vi "TagDB Refresh UI Value.vi"() -> ()   [LabVIEW 2017]
uses:
  2ef29265-346b-4d57-9e06-764a04e9d281.vi
  f314512e-c22b-4d02-bdf1-59be9bdd757c.vi
  22528161-74fa-4c81-9678-da9be87c1aa3.vi
  8fbe6154-e4cc-4ea5-b8fc-074bb6443d9f.vi
  f2742c4f-3dd1-44df-a39f-d6b0d834631b.vi
  922adba5-6730-477c-a9a6-f6ae257f51b2.vi
  c4b4571f-6e89-4cba-b3ba-78e7cbfa36bb.vi
  TagDB/_Support/DataAccess/data-Write.vi
  TagDB/_Support/Error/_[error50000]Invalid DB REF.vi
  TagDB/_Support/DataAccess/TagDB Ref to DVR.vi
  TagDB/_Support/DataAccess/_NameCacher.vi
  TagDB/_Support/Error/_[error50002]Invalid DataType.vi
  TagDB/_Support/URL/TRIM-BOTH-SPACE.vi
  TagDB/_Support/DataAccess/_datatypeChecker.vi
  <vilib>/Utility/Data Type/Get Type Information.vi
  TagDB/_Support/Error/_Build Error Cluster.vi
  TagDB/TagDB.lvlib
panel:
  in  "Update Period(ms)":u32(slide)=100 scale=1.0..1000.0
  out "String":string
  out "Numeric":dbl
  in  "stop":bool
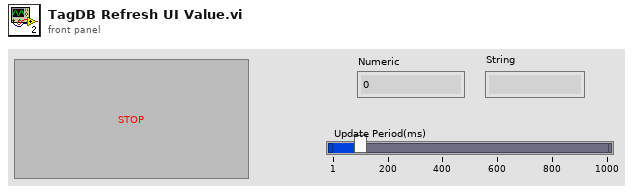
[diagram p1: front panel]
types:
  T1 = typedef "TagDB.lvlib/TagDB.ctl" = refnum<k1>
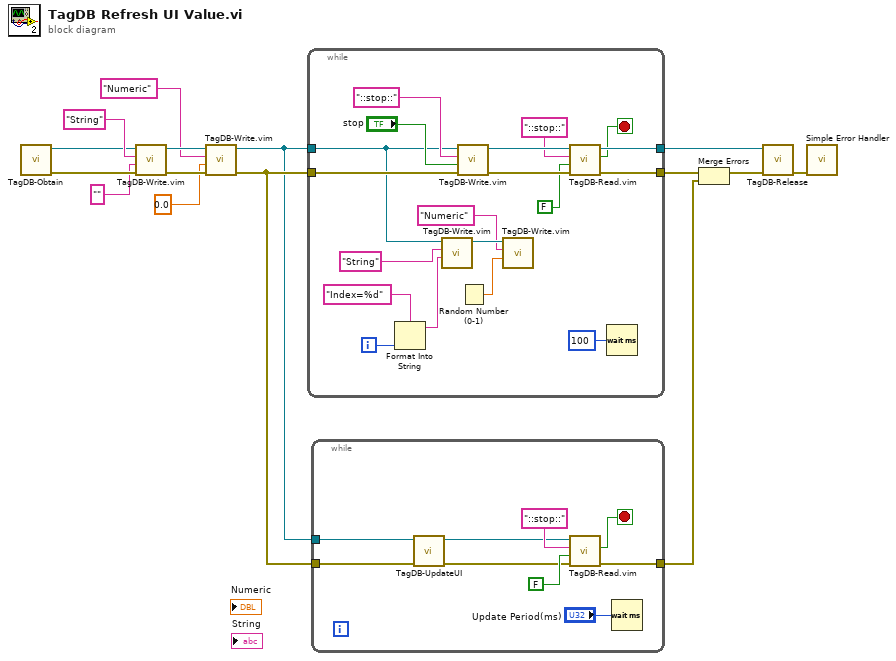
[diagram p0: block diagram]
diagram:
  n1 = call "TagDB-Obtain.vi"() -> ("error out"=w10:errorcluster, "TagDB"=w11:T1)  [unwired: 5 in, 1 out]
  n2 = call "TagDB-Write.vim"("error in (no error)"=w10, "Value"="" ("String"), "tag"="String" ("String"), "TagDB"=w11) -> ("error out"=w7:errorcluster, "TagDB(dup)"=w5:T1)  [unwired: 5 in, 1 out]
  n3 = call "TagDB-Write.vim"("error in (no error)"=w7, "Value"=0.0, "tag"="Numeric" ("String"), "TagDB"=w5) -> ("error out"=w6:errorcluster, "TagDB(dup)"=w4:T1)  [unwired: 5 in, 1 out]
  n4 = while {
    tunnel: w4 -> [w19]
    tunnel: w6 -> [w33]
    tunnel: [w26] -> w9
    tunnel: [w29] -> w14
    i -> [w23]
    stop <- w25 stop-if-true
    n5 = Format Into String(format string="Index=%d", w23) -> (resulting string=w20:string)  [unwired: 2 in, 1 out]
    n6 = call "TagDB-Write.vim"("Value"=w20, "tag"="String" ("String"), "TagDB"=w19) -> ("TagDB(dup)"=w18:T1)  [unwired: 6 in, 2 out]
    n7 = call "TagDB-Write.vim"("error in (no error)"=w33, "Value"="stop", "tag"="::stop::" ("name"), "TagDB"=w19) -> ("error out"=w27:errorcluster, "TagDB(dup)"=w30:T1)  [unwired: 5 in, 1 out]
    n8 = Random Number (0-1)() -> (number: 0 to 1=w16:dbl)
    n9 = call "TagDB-Write.vim"("Value"=w16, "tag"="Numeric" ("String"), "TagDB"=w18) -> ()  [unwired: 6 in, 3 out]
    n10 = call "TagDB-Read.vim"("error in (no error)"=w27, "Type(empty to read as variant)"=FALSE, "name"="::stop::", "TagDB"=w30) -> ("error out"=w26:errorcluster, "Value"=w25:bool, "TagDB(dup)"=w29:T1)  [unwired: 2 in, 3 out]
    n11 = Wait (ms)(milliseconds to wait=u32 100) -> ()  [unwired: 1 out]
  }
  n12 = while {
    tunnel: w4 -> [w38]
    tunnel: w6 -> [w37]
    tunnel: [w41] -> w8
    stop <- w40 stop-if-true
    n13 = call "TagDB-UpdateUI.vi"("error in (no error)"=w37, "TagDB"=w38) -> ("error out"=w36:errorcluster, "TagDB(dup)"=w35:T1)  [unwired: 8 in]
    n14 = call "TagDB-Read.vim"("error in (no error)"=w36, "Type(empty to read as variant)"=FALSE, "name"="::stop::", "TagDB"=w35) -> ("error out"=w41:errorcluster, "Value"=w40:bool)  [unwired: 2 in, 4 out]
    n15 = Wait (ms)(milliseconds to wait="Update Period(ms)") -> ()  [unwired: 1 out]
  }
  n16 = Merge Errors(w9, w8) -> (w13:errorcluster)
  n17 = call "TagDB-Release.vi"("error in (no error)"=w13, "TagDB"=w14) -> ("error out"=w15:errorcluster)  [unwired: 9 in]
  n18 = call <vilib>:"Simple Error Handler.vi"("error in (no error)"=w15) -> ()  [unwired: 4 in, 5 out]
